vi "Facade.vi"(0 "Data In":T4, 2 "Display State In":T2, 3 "Container State":T3) -> (6 "Data Out":T4, 7 "Display State Out":T2, 8 "Action":T1)   [LabVIEW 2020, in "Level (G3).xctl"]
uses:
  Level (G3).xctl
  Level Data.ctl
  Level Units (G3).ctl
  <vilib>/_xctls/Container State.ctl
  State.ctl
  Utility VIs/Controls/KRing/KRing.xctl
  Utility VIs/Controls/KNumeric (DBL)/KNumeric (DBL).xctl
  <vilib>/_xctls/Action.ctl
  <vilib>/_xctls/XControlSupport.lvlib
panel:
  out "display state signal":bool
  in  "Refresh Button":bool
  out "Max":dbl
  in  "Units":i16(xcontrol)
  in  "Level":dbl(xcontrol)
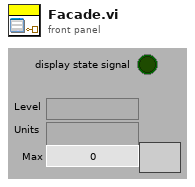
[diagram p1: front panel]
types:
  T1 = typedef "XControlSupport.lvlib/Action.ctl" = cluster{"Data Changed?":bool, "State Changed?":bool, "Action Name":string}
  T2 = typedef "Level (G3).xctl/State.ctl" = cluster{"LMax Event":refnum<user-event>, "enable menu":bool, "Units":string[], "Valid":bool[], "multi":bool, "ctl":cluster{"Units":refnum<vi>, "Level":refnum<vi>}}
  T3 = typedef "XControlSupport.lvlib/Container State.ctl" = cluster{"Indicator?":bool, "Run Mode?":bool, " Refnum":refnum<vi>}
  T4 = typedef "Level (G3).xctl/Level Data.ctl" = cluster{"Level":dbl, "Units":T5, "Max":dbl, "Data":cluster{"Multiplier":dbl, "Cal File":path, "Cal":cluster{"Freq (Hz)":dbl[], "Mag (dB SPL)":dbl[], "Phase (deg)":dbl[]}, "audiogram":path}}
  T5 = typedef "Level (G3).xctl/Level Units (G3).ctl" = enum16{"dB atten", "dB SPL", "dB re 1 Vrms", "dB V/Hz½", "mW", "dB HL", "Volts", "dB mW"}
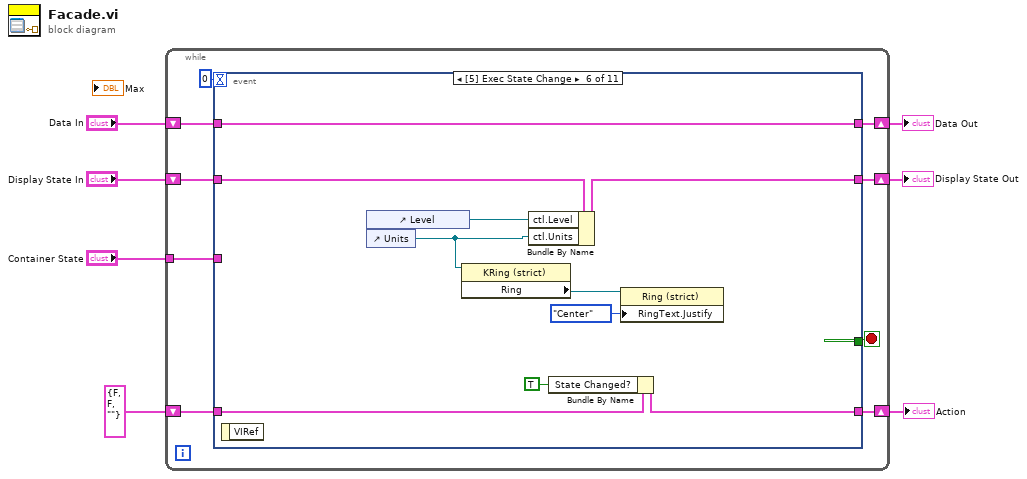
[diagram p0: block diagram]
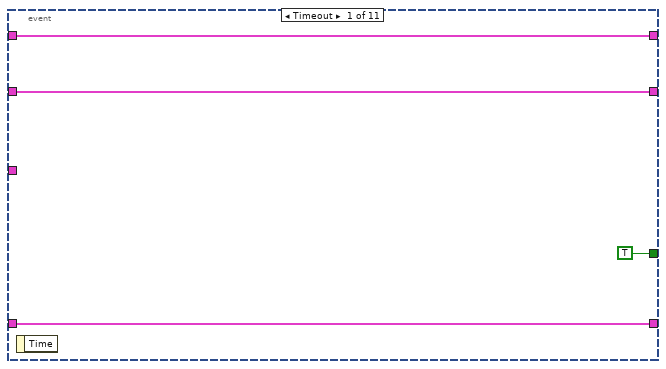
[diagram p2: hidden frame]
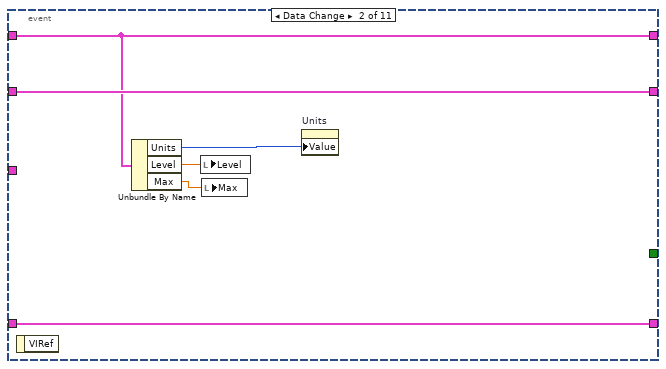
[diagram p3: hidden frame]
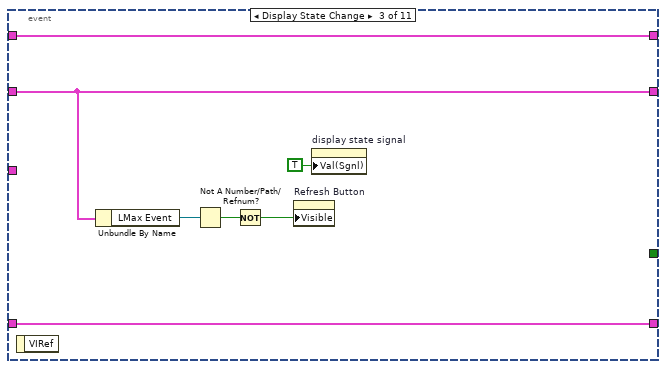
[diagram p4: hidden frame]
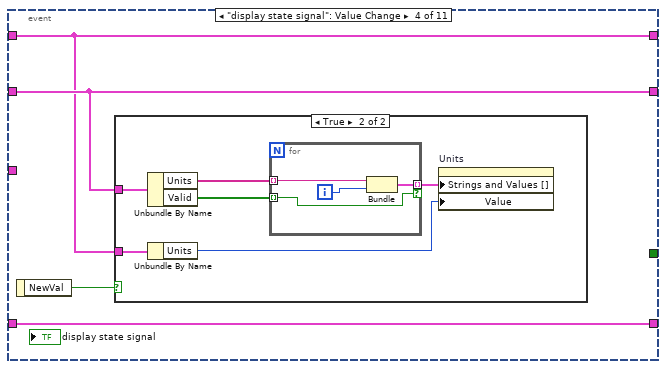
[diagram p5: hidden frame]
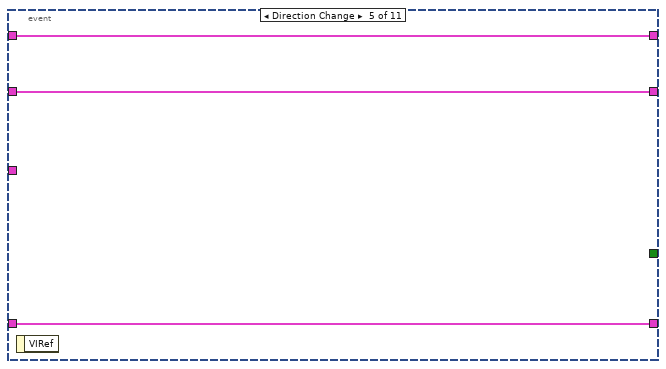
[diagram p7: hidden frame]
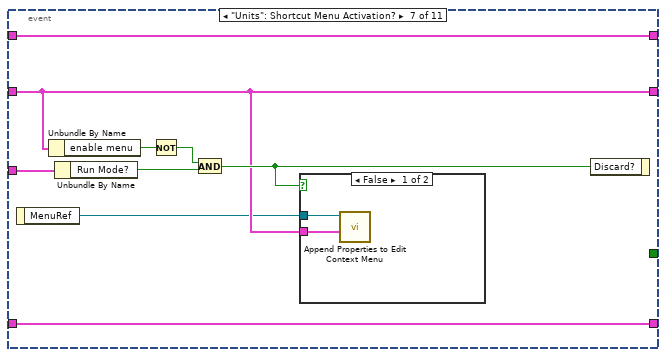
[diagram p8: hidden frame]
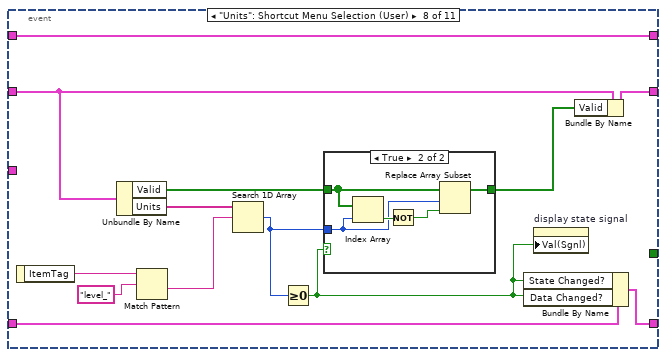
[diagram p10: hidden frame]
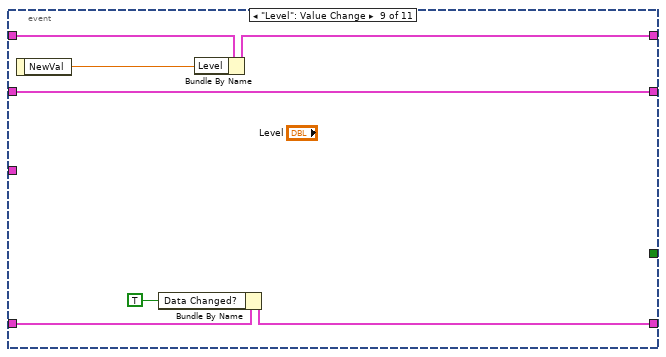
[diagram p12: hidden frame]
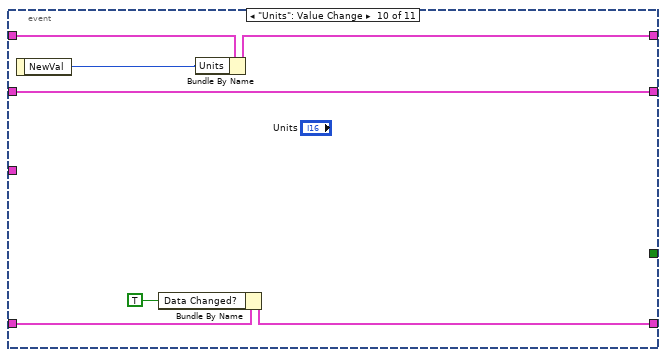
[diagram p13: hidden frame]
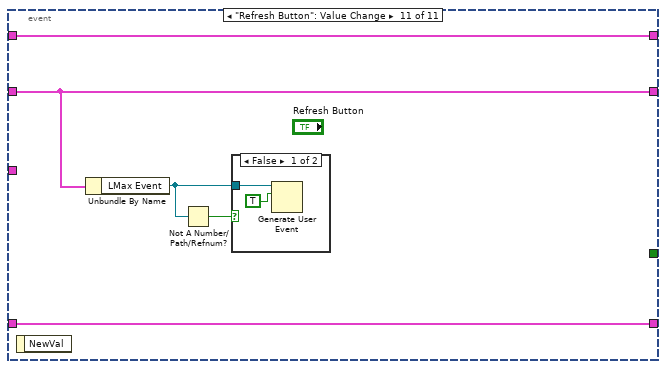
[diagram p14: hidden frame]
diagram:
  n1 = while {
    shift-right: [w15] -> w4
    shift-left: "Display State In" -> [w16]
    tunnel: "Container State" -> [w12]
    shift-right: [w10] -> w7
    shift-left: "Data In" -> [w11]
    shift-right: [w8] -> w2
    shift-left: T1 {"Data Changed?"=FALSE, "State Changed?"=FALSE, "Action Name"=""} ("Action") -> [w9]
    stop <- w14 stop-if-true
    n2 = event shown="[5] Exec State Change" {
      selector: _ -> [_ _ _ _ _ _ _ _ _ _ _]
      dyn-events: _ -> [_ _ _ _ _ _ _ _ _ _ _]
      timeout: 0 -> [_ _ _ _ _ _ _ _ _ _ _]
      tunnel: w16 -> [w18 w26 w30 w36 w50 w60 w62 w73 w91 w98 w107]
      tunnel: [w18 w26 w30 w36 w50 w57 w62 w78 w91 w98 w107] -> w15
      tunnel: [TRUE _ _ _ _ _ _ _ _ _ _] -> w14
      tunnel: w12 -> [_ _ _ _ _ _ w64 _ _ _ _]
      tunnel: w11 -> [w17 w24 w33 w34 w49 w59 w69 w84 w97 w104 w109]
      tunnel: [w17 w24 w33 w34 w49 w59 w69 w84 w95 w102 w109] -> w10
      tunnel: [w19 w25 w32 w37 w48 w56 w68 w79 w92 w99 w108] -> w8
      tunnel: w9 -> [w19 w25 w32 w37 w48 w58 w68 w80 w94 w101 w108]
      event Timeout {
        n3 = event-data() -> ()  [unwired: 1 in, 1 out]
      }
      event Data Change {
        n4 = event-data() -> ()  [unwired: 1 in, 1 out]
        n5 = Unbundle By Name(w24) -> ("Units"=w21:T5, "Level"=w23:dbl, "Max"=w22:dbl)
        n6 = local write "Level"(w23) -> ()
        n7 = local write "Max"(w22) -> ()
        n8 = property on="Units" class="KRing (strict)"("Value"=w21) -> ()  [unwired: 2 in, 2 out]
      }
      event Display State Change {
        n9 = event-data() -> ()  [unwired: 1 in, 1 out]
        n10 = Unbundle By Name(w30) -> ("LMax Event"=w29:refnum<user-event>)
        n11 = Not A Number/Path/Refnum?(number/path/refnum=w29) -> (NaN/Path/Refnum?=w28:bool)
        n12 = Not(x=w28) -> (.not. x?=w27:bool)
        n13 = property on="Refresh Button" class="Bool"("Visible"=w27) -> ()  [unwired: 2 in, 2 out]
        n14 = property on="display state signal" class="Bool (strict)"("Val(Sgnl)"=TRUE ("Value (Signaling)")) -> ()  [unwired: 2 in, 2 out]
      }
      event "display state signal": Value Change {
        n15 = event-data() -> ("NewVal"=w35:bool)  [unwired: 1 in]
        n16 = case shown="True" w35 {
          tunnel: w36 -> [_ w40]
          tunnel: w34 -> [_ w39]
          frame False {
          }
          frame True {
            n17 = Unbundle By Name(w40) -> ("Units"=w42:string[], "Valid"=w43:bool[])
            n18 = Unbundle By Name(w39) -> ("Units"=w38:T5)
            n19 = for {
              tunnel: w43 -> [w44] mode=indexing
              tunnel: w42 -> [w45] mode=indexing
              tunnel: [w47] -> w41 mode=indexing if=w44
              i -> [w46]
              n20 = Bundle("String"=w45, w46) -> (w47:cluster{"String":string, i32})  [unwired: 1 in]
            }
            n21 = property on="Units" class="KRing (strict)"("Strings and Values []"=w41, "Value"=w38) -> ()  [unwired: 2 in, 2 out]
          }
        }
      }
      event Direction Change {
        n22 = event-data() -> ()  [unwired: 1 in, 1 out]
      }
      event Exec State Change {
        n23 = event-data() -> ()  [unwired: 1 in, 1 out]
        n24 = control-ref of="Level"() -> (w54:refnum<vi>)
        n25 = control-ref of="Units"() -> (w53:refnum<vi>)
        n26 = property class="KRing (strict)"(reference=w53) -> ("Ring"=w52:refnum<vi>)  [unwired: 1 in, 2 out]
        n27 = Bundle By Name(cluster=w60, "ctl.Level"=w54, "ctl.Units"=w53) -> (w57:T2)
        n28 = Bundle By Name(cluster=w58, "State Changed?"=TRUE) -> (w56:T1)
        n29 = property class="Ring (strict)"(reference=w52, "RingText.Justify"=enum16{"Left", "Center", "Right"}."Center" ("Ring Text.Justification")) -> ()  [unwired: 1 in, 2 out]
      }
      event "Units": Shortcut Menu Activation? {
        n30 = event-data() -> ("MenuRef"=w61:refnum<k9>)  [unwired: 1 in]
        n31 = Unbundle By Name(w62) -> ("enable menu"=w66:bool)
        n32 = Unbundle By Name(w64) -> ("Run Mode?"=w65:bool)
        n33 = Not(x=w66) -> (.not. x?=w67:bool)
        n34 = And(x=w67, y=w65) -> (x .and. y?=w63:bool)
        n35 = case shown="False" w63 {
          tunnel: w62 -> [w70 _]
          tunnel: w61 -> [w71 _]
          frame False {
            n36 = call "Append Properties to Edit Context Menu.vi"("State"=w70, "Menu in"=w71) -> ()  [unwired: 10 in]
          }
          frame True {
          }
        }
        n37 = event-data("Discard?"=w63) -> ()  [unwired: 1 in, 1 out]
      }
      event "Units": Shortcut Menu Selection (User) {
        n38 = event-data() -> ("ItemTag"=w75:string)  [unwired: 1 in]
        n39 = Unbundle By Name(w73) -> ("Valid"=w82:bool[], "Units"=w81:string[])
        n40 = Match Pattern(string=w75, regular expression="level_" ("string")) -> (after substring=w76:string)  [unwired: 1 in, 3 out]
        n41 = Search 1D Array(1D array=w81, element=w76) -> (index of element=w83:i32)  [unwired: 1 in]
        n42 = Greater Or Equal To 0?(x=w83) -> (x >= 0?=w72:bool)
        n43 = case shown="True" w72 {
          tunnel: w82 -> [w85 w88]
          tunnel: w83 -> [_ w86]
          tunnel: [w85 w87] -> w77
          frame False {
          }
          frame True {
            n44 = Index Array(array=w88, index=w86) -> (element=w90:bool)
            n45 = Not(x=w90) -> (.not. x?=w89:bool)
            n46 = Replace Array Subset(array=w88, new element=w89, index=w86) -> (w87:bool[])
          }
        }
        n47 = Bundle By Name(cluster=w80, "State Changed?"=w72, "Data Changed?"=w72) -> (w79:T1)
        n48 = property on="display state signal" class="Bool (strict)"("Val(Sgnl)"=w72) -> ()  [unwired: 2 in, 2 out]
        n49 = Bundle By Name(cluster=w73, "Valid"=w77) -> (w78:T2)
      }
      event "Level": Value Change {
        n50 = event-data() -> ("NewVal"=w96:dbl)  [unwired: 1 in]
        n51 = Bundle By Name(cluster=w94, "Data Changed?"=TRUE) -> (w92:T1)
        n52 = Bundle By Name(cluster=w97, "Level"=w96) -> (w95:T4)
      }
      event "Units": Value Change {
        n53 = event-data() -> ("NewVal"=w103:i16)  [unwired: 1 in]
        n54 = Bundle By Name(cluster=w101, "Data Changed?"=TRUE) -> (w99:T1)
        n55 = Bundle By Name(cluster=w104, "Units"=w103) -> (w102:T4)
      }
      event "Refresh Button": Value Change {
        n56 = event-data() -> ()  [unwired: 1 in, 1 out]
        n57 = Unbundle By Name(w107) -> ("LMax Event"=w105:refnum<user-event>)
        n58 = Not A Number/Path/Refnum?(number/path/refnum=w105) -> (NaN/Path/Refnum?=w106:bool)
        n59 = case shown="False" w106 {
          tunnel: w105 -> [w111 _]
          frame False {
            n60 = Generate User Event(user event=w111, event data cluster=TRUE) -> ()  [unwired: 2 in, 2 out]
          }
          frame True {
          }
        }
      }
    }
  }
  "Display State Out" <- w4
  "Data Out" <- w7
  "Action" <- w2
